vi "Config Spindle.vi"(0 "Maximum spindle speed\tRPM":u32, 5 "Minimum spindle speed\tRPM":u32, 11 "error in (no error)":errorcluster) -> (15 "error out":errorcluster)   [LabVIEW 2024, in "GRBL 1.1.lvlib"]
doc: "Maximum spindle speed RPM: Maximum spindle speed. Sets PWM to 100% duty cycle.\nMinimum spindle speed RPM: Minimum spindle speed. Sets PWM to 0.4% or lowest duty cycle."
uses:
  GRBL 1.1.lvlib
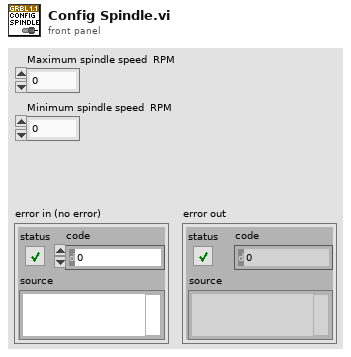
[diagram p1: front panel]
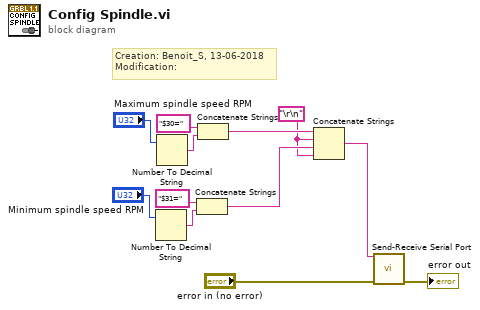
[diagram p0: block diagram]
diagram:
  w2 = "\r\n"
  # "Creation: Benoit_S, 13-06-2018\nModification:"
  n1 = Number To Decimal String(number="Minimum spindle speed\tRPM") -> (decimal integer string=w7:string)  [unwired: 1 in]
  n2 = Number To Decimal String(number="Maximum spindle speed\tRPM") -> (decimal integer string=w10:string)  [unwired: 1 in]
  n3 = Concatenate Strings("$31=", w7) -> (w3:string)
  n4 = Concatenate Strings("$30=", w10) -> (w4:string)
  n5 = Concatenate Strings(w4, w2, w3, w2) -> (w1:string)
  n6 = call "Send-Receive Serial Port.vi"("Data to write"=w1, "error in (no error)"="error in (no error)") -> ("error out"=→"error out":errorcluster)  [unwired: 12 in, 1 out]
